vi "Main smart home.vi"() -> ()   [LabVIEW 2016]
uses:
  Typedef/Serial_config_cluster.ctl
panel:
  in  "Send string to MCU":bool
  in  "Analyse":bool
  out "STOP ALL Indicator 2":bool
  in  "STOP ALL":bool
  in  "STOP ALL 2":bool
  out "Button Chooser Online":bool
  out "STOP ALL Indicator":bool
  in  "Settings Button":bool
  in  "Open Led control":bool
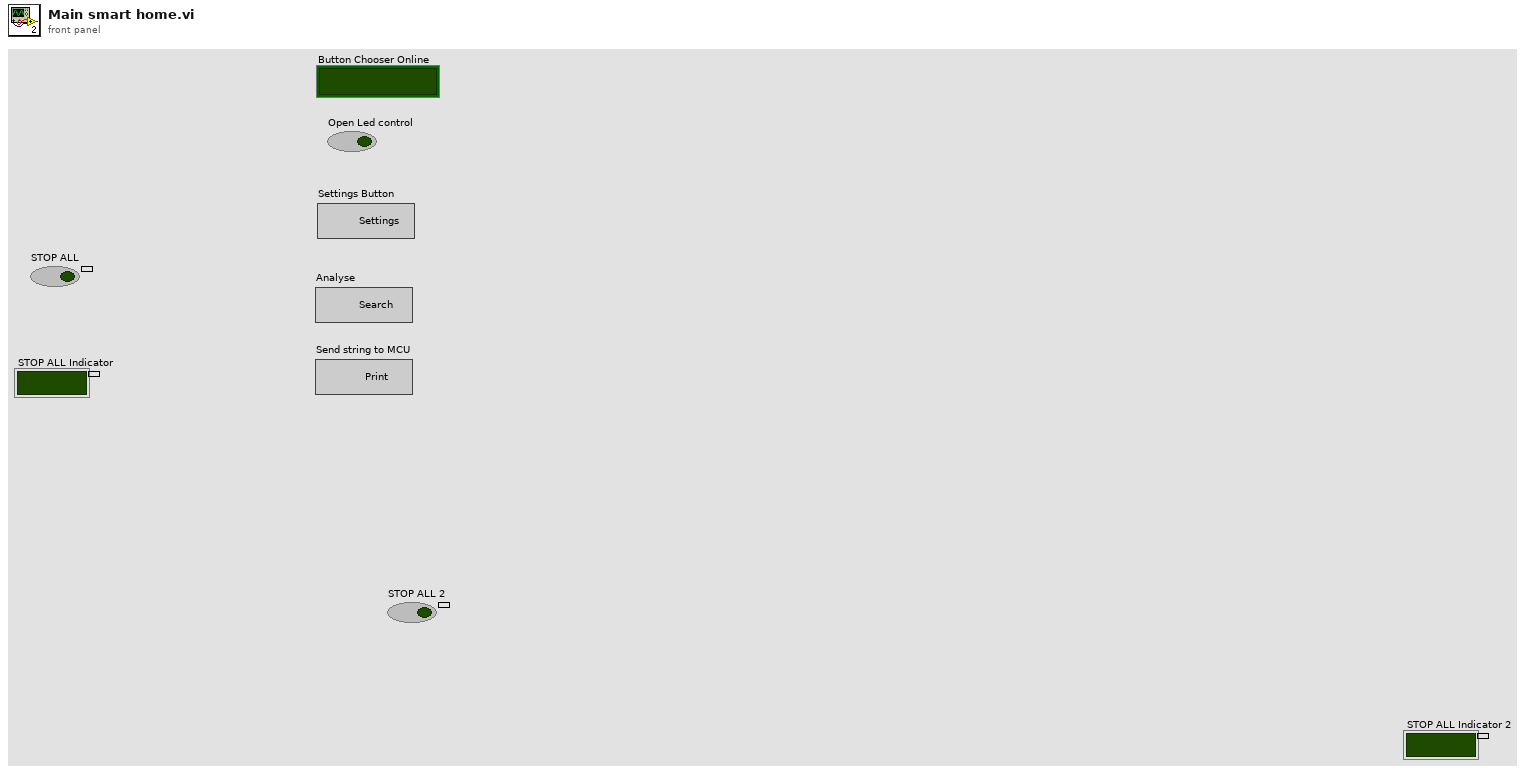
[diagram p1: front panel]
types:
  T1 = typedef "Serial_config_cluster.ctl" = cluster{"Termination Character":u8, "End Read on":bool, "VISA resource name":refnum<visa-resource-name>, "baud rate":u32, "data bits":u16, "parity":enum16{"None", "Odd", "Even", "Mark", "Space"}, "stop bits":u16, "flow control":u16, "XON":enum16{"NUL", "SOH", "STX", "ETX", "EOT", "ENQ", "ACK", "BEL", "BS", "HT", "LF", "VT", "FF", "CR", "SO", "SI", "DLE", "DC1", "DC2", "DC3", "DC4", "NAK", "SYN", "ETB", "CAN", "EM", "SUB", "ESC", "FS", "GS", "RS", "US", "SP", "!", "\"", "#", "$", "%", "&", "'", "(", ")", "*", "+", ",", "- (-)", ".", "/", "0", "1", "2", "3", "4", "5", "6", "7", "8", "9", ":", ";", "<", "=", ">", "?", "@", "A", "B", "C", "D", "E", "F", "G", "H", "I", "J", "K", "L", "M", "N", "O", "P", "Q", "R", "S", "T", "U", "V", "W", "X", "Y", "Z", "[", "\\", "]", "^", "_", "`", "a", "b", "c", "d", "e", "f", "g", "h", "i", "j", "k", "l", "m", "n", "o", "p", "q", "r", "s", "t", "u", "v", "w", "x", "y", "z", "{", "|", "}", "~"}, "XOFF":enum16{"NUL", "SOH", "STX", "ETX", "EOT", "ENQ", "ACK", "BEL", "BS", "HT", "LF", "VT", "FF", "CR", "SO", "SI", "DLE", "DC1", "DC2", "DC3", "DC4", "NAK", "SYN", "ETB", "CAN", "EM", "SUB", "ESC", "FS", "GS", "RS", "US", "SP", "!", "\"", "#", "$", "%", "&", "'", "(", ")", "*", "+", ",", "- (-)", ".", "/", "0", "1", "2", "3", "4", "5", "6", "7", "8", "9", ":", ";", "<", "=", ">", "?", "@", "A", "B", "C", "D", "E", "F", "G", "H", "I", "J", "K", "L", "M", "N", "O", "P", "Q", "R", "S", "T", "U", "V", "W", "X", "Y", "Z", "[", "\\", "]", "^", "_", "`", "a", "b", "c", "d", "e", "f", "g", "h", "i", "j", "k", "l", "m", "n", "o", "p", "q", "r", "s", "t", "u", "v", "w", "x", "y", "z", "{", "|", "}", "~"}, "End Write on":bool}
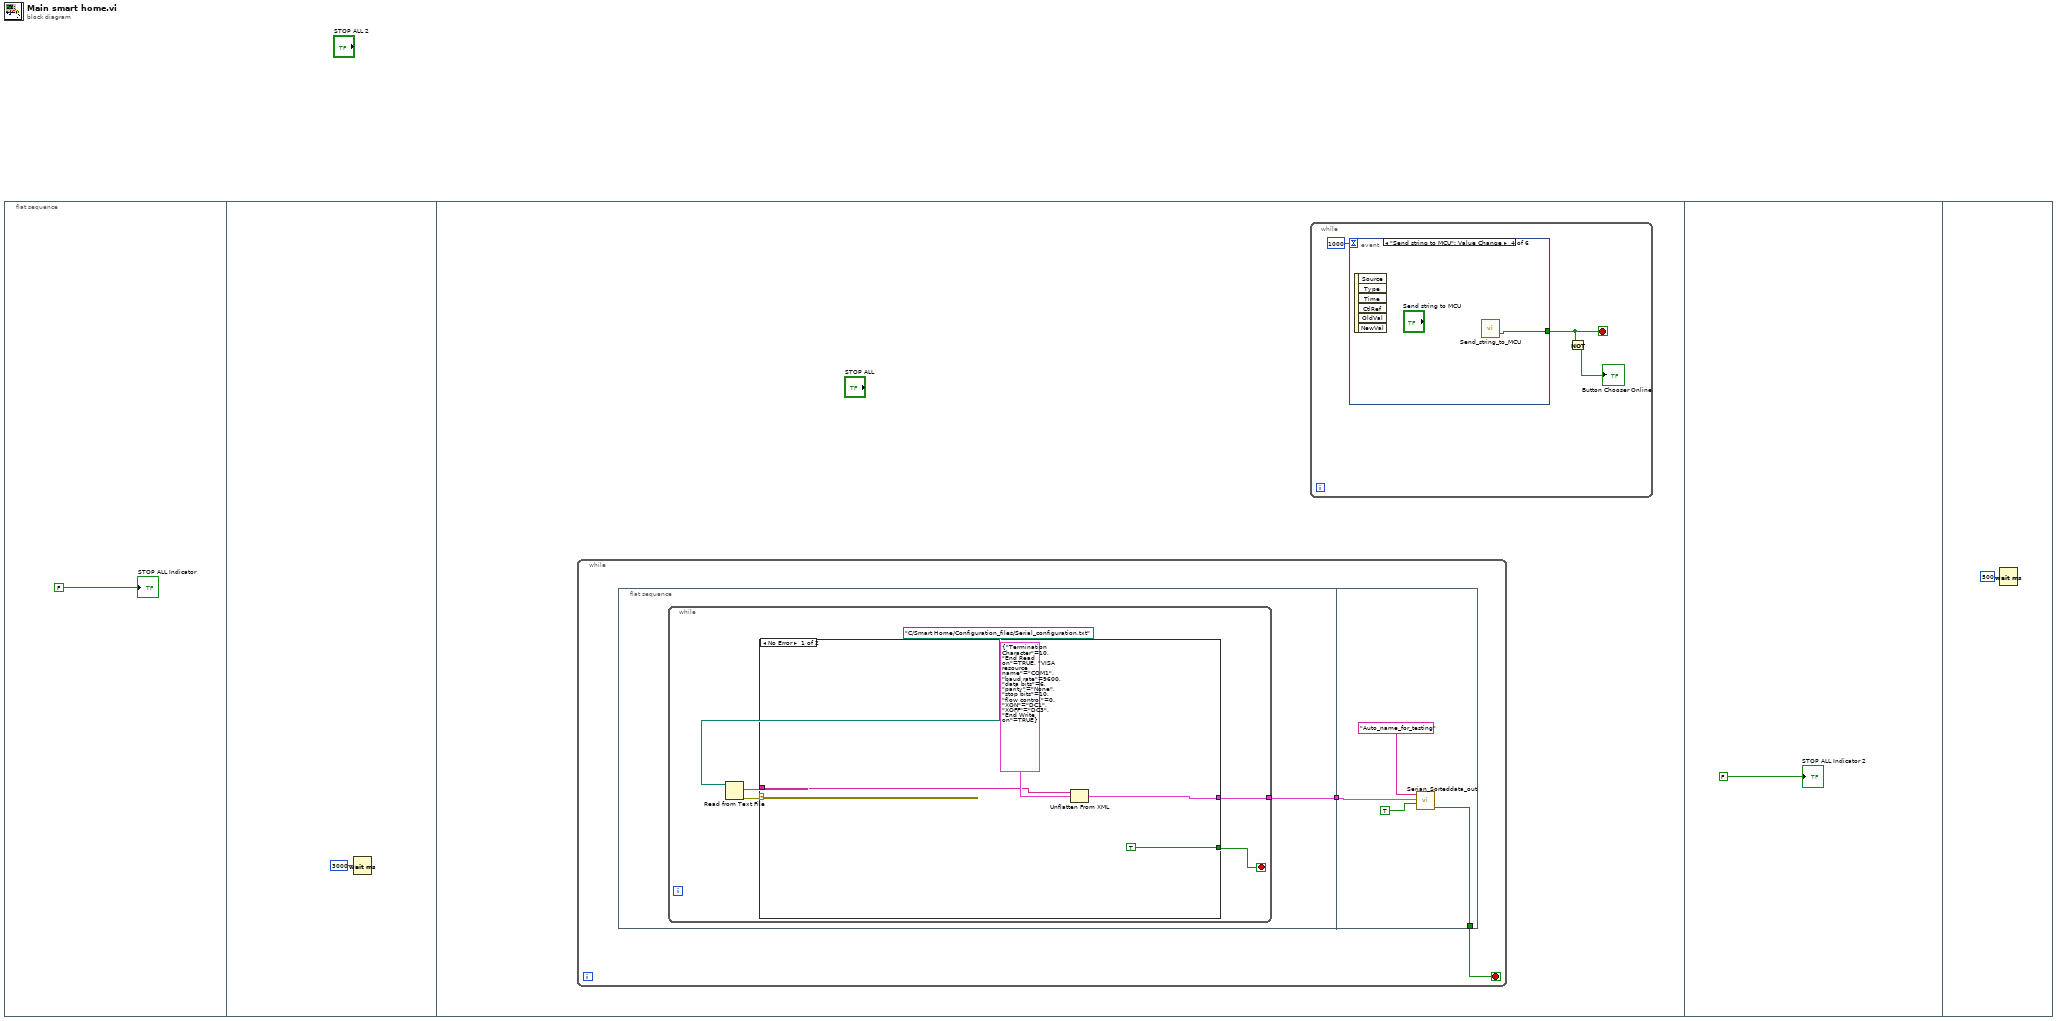
[diagram p0: block diagram]
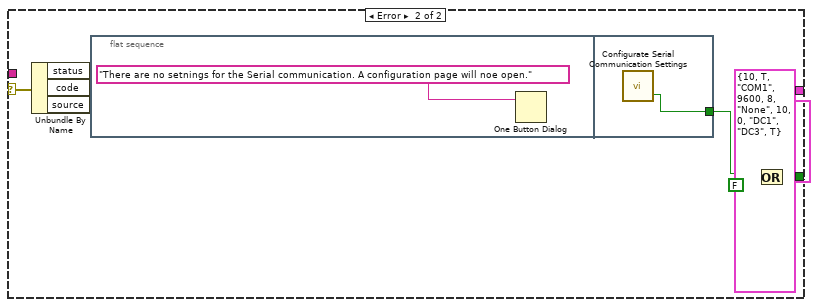
[diagram p2: hidden frame]
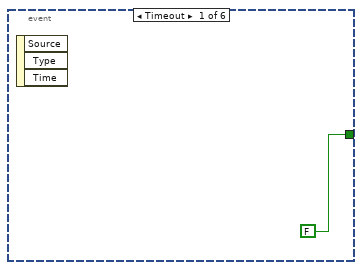
[diagram p3: hidden frame]
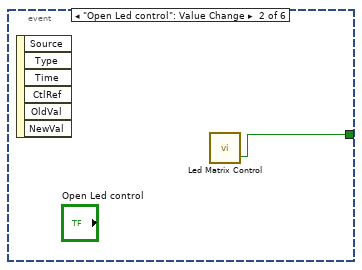
[diagram p4: hidden frame]
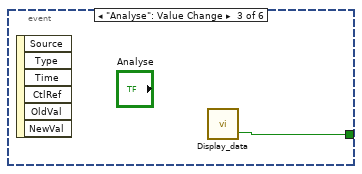
[diagram p5: hidden frame]
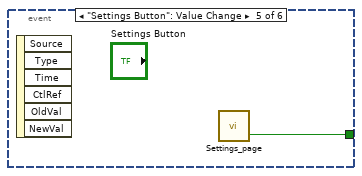
[diagram p6: hidden frame]
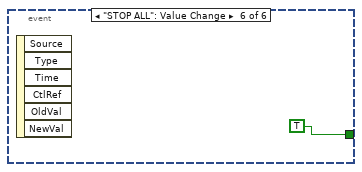
[diagram p7: hidden frame]
diagram:
  n1 = flat-sequence {
    frame #0 {
      "STOP ALL Indicator" <- FALSE ("STOP ALL")
    }
    frame #1 {
      n2 = Wait (ms)(milliseconds to wait=u32 3000) -> ()  [unwired: 1 out]
    }
    frame #2 {
      n3 = while {
        stop <- w3 stop-if-true
        n4 = flat-sequence {
          tunnel: [w5] -> w4
          tunnel: w4 -> [w24]
          tunnel: [w23] -> w3
          frame #0 {
            n5 = while {
              tunnel: [w7] -> w5
              stop <- w6 stop-if-true
              n6 = Read from Text File(file (use dialog)=path "C:/Smart Home/Configuration_files/Serial_configuration.txt") -> (text=w9:string, error out=w8:errorcluster)  [unwired: 3 in, 2 out]
              n7 = case shown="No Error" w8 {
                selector: w8 -> [_ w19]
                tunnel: w9 -> [w13 _]
                tunnel: [w12 T1 {"Termination Character"=10, "End Read on"=TRUE, "VISA resource name"="COM1", "baud rate"=9600, "data bits"=8, "parity"=enum."None", "stop bits"=10, "flow control"=0, "XON"=enum."DC1", "XOFF"=enum."DC3", "End Write on"=TRUE} ("Cluster 2")] -> w7
                tunnel: [TRUE w17] -> w6
                frame No Error {
                  n8 = Unflatten From XML(xml string=w13, type=T1 {"Termination Character"=10, "End Read on"=TRUE, "VISA resource name"="COM1", "baud rate"=9600, "data bits"=6, "parity"=enum."None", "stop bits"=10, "flow control"=0, "XON"=enum."DC1", "XOFF"=enum."DC3", "End Write on"=TRUE} ("Cluster 2")) -> (value=w12:T1)  [unwired: 1 in, 1 out]
                }
                frame Error {
                  n9 = Unbundle By Name(w19) -> ()  [unwired: 3 out]
                  n10 = flat-sequence {
                    tunnel: [w21] -> w15
                    frame #0 {
                      n11 = One Button Dialog(message="There are no setnings for the Serial communication. A configuration page will noe open.") -> ()  [unwired: 1 in, 1 out]
                    }
                    frame #1 {
                      n12 = call "Configurate Serial Communication Settings.vi"() -> ("STOP ALL 2"=w21:bool)  [unwired: 2 in, 1 out]
                    }
                  }
                  n13 = Or(x=w15, y=FALSE) -> (x .or. y?=w17:bool)
                }
              }
            }
          }
          frame #1 {
            n14 = call "Serian_Sorteddata_out.vi"("Save"=TRUE, "Cluster"=w24, "File_name"="Auto_name_for_testing") -> ("MAIN STOP OUT"=w23:bool)  [unwired: 8 in]
          }
        }
      }
      n15 = while {
        stop <- w28 stop-if-true
        n16 = event shown="[3] \"Send string to MCU\": Value Change" {
          selector: _ -> [_ _ _ _ _ _]
          dyn-events: _ -> [_ _ _ _ _ _]
          timeout: 1000 -> [_ _ _ _ _ _]
          tunnel: [FALSE ("NewVal") w30 w31 w32 w33 TRUE] -> w28
          event Timeout {
            n17 = event-data() -> ()  [unwired: 1 in, 3 out]
          }
          event "Open Led control": Value Change {
            n18 = event-data() -> ()  [unwired: 1 in, 6 out]
            n19 = call "Led Matrix Control.vi"() -> ("STOP ALL OUT"=w30:bool)  [unwired: 3 in]
          }
          event "Analyse": Value Change {
            n20 = event-data() -> ()  [unwired: 1 in, 6 out]
            n21 = call "Display_data.vi"() -> ("STOP ALL 2"=w31:bool)  [unwired: 3 in]
          }
          event "Send string to MCU": Value Change {
            n22 = event-data() -> ()  [unwired: 1 in, 6 out]
            n23 = call "Send_string_to_MCU.vi"() -> ("STOP ALL 2"=w32:bool)  [unwired: 3 in]
          }
          event "Settings Button": Value Change {
            n24 = event-data() -> ()  [unwired: 1 in, 6 out]
            n25 = call "Settings_page.vi"() -> ("STOP ALL OUT"=w33:bool)  [unwired: 3 in]
          }
          event "STOP ALL": Value Change {
            n26 = event-data() -> ()  [unwired: 1 in, 6 out]
          }
        }
        n27 = Not(x=w28) -> (.not. x?=→"Button Chooser Online":bool)
      }
    }
    frame #3 {
      "STOP ALL Indicator 2" <- FALSE ("STOP ALL")
    }
    frame #4 {
      n28 = Wait (ms)(milliseconds to wait=u32 500) -> ()  [unwired: 1 out]
    }
  }
